vi "BELLA PW scan mode shot control shutter.vi"(8 "error in (no error)":errorcluster, 10 "PostScanRate":dbl=0.006 min=-9999999.0 max=9999999.0 format="%#_3f", 11 "ScanShotControl":bool) -> (0 "error out":errorcluster, 3 "delay D to set":dbl)   [LabVIEW 2020]
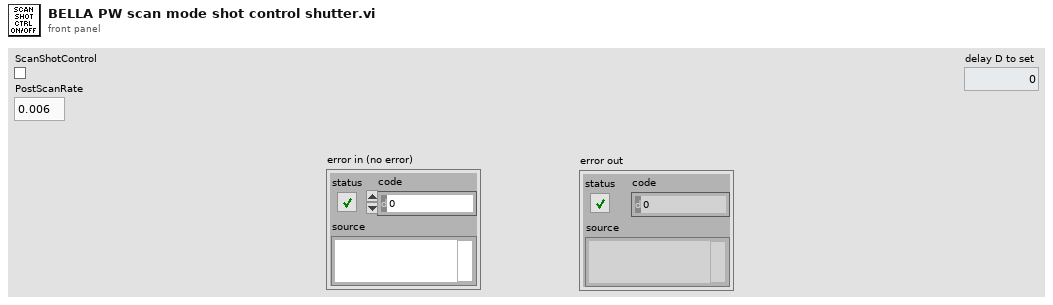
[diagram p1: front panel]
types:
  T1 = typedef "mysql_authentication.ctl" = cluster{"User":string, "Password":string, "Database":string}
  T2 = cluster{"Port":u16, "IP Address":string, "Authentication":T1}
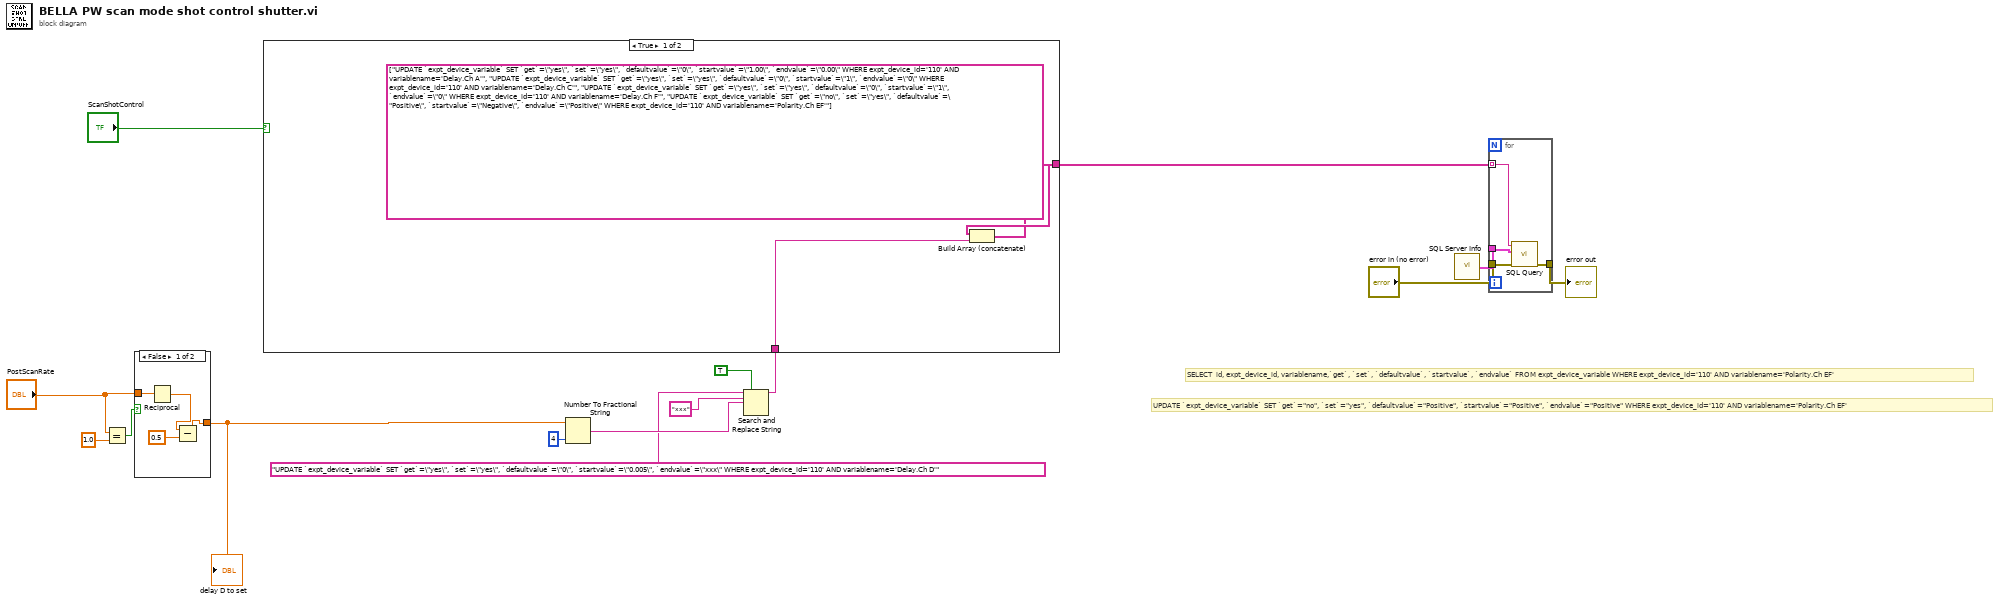
[diagram p0: block diagram]
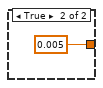
[diagram p2: hidden frame]
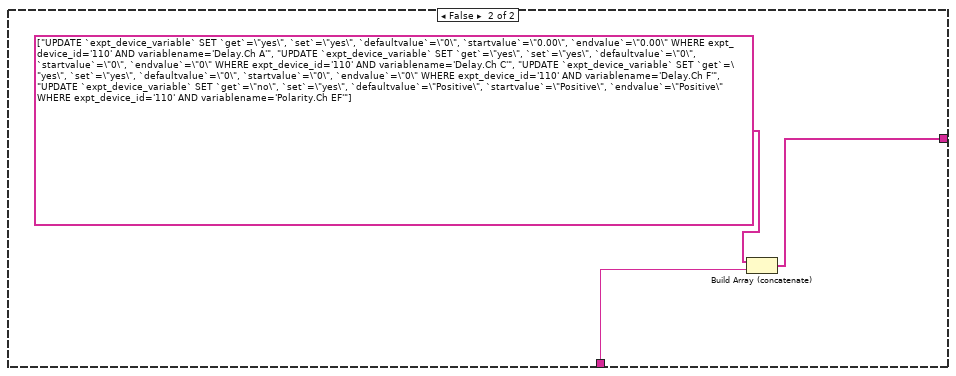
[diagram p3: hidden frame]
diagram:
  # "UPDATE `expt_device_variable` SET `get`=\"no\", `set`=\"yes\", `defaultvalue`=\"Positive\", `startvalue`=\"Positive\", `endvalue`=\"Positive\" WHERE expt_device_id='110' AND variablename='Polarity.Ch EF'"
  # "SELECT  id, expt_device_id, variablename,`get`, `set`, `defaultvalue`, `startvalue`, `endvalue` FROM expt_device_variable WHERE expt_device_id='110' AND variablename='Polarity.Ch EF'"
  n1 = Equal?(x="PostScanRate", y=1.0) -> (x = y?=w8:bool)
  n2 = case shown="False" w8 {
    tunnel: "PostScanRate" -> [w19 _]
    tunnel: [w16 0.005 ("y")] -> w5
    frame False {
      n3 = Reciprocal(x=w19) -> (1/x=w18:dbl)
      n4 = Subtract(x=w18, y=0.5) -> (x-y=w16:dbl)
    }
    frame True {
    }
  }
  "delay D to set" <- w5
  n5 = Number To Fractional String(number=w5, precision (6)=i16 4) -> (F-format string=w7:string)  [unwired: 2 in]
  n6 = Search and Replace String(replace all?=TRUE ("replace all? (F)"), input string="UPDATE `expt_device_variable` SET `get`=\"yes\", `set`=\"yes\", `defaultvalue`=\"0\", `startvalue`=\"0.005\", `endvalue`=\"xxx\" WHERE expt_device_id='110' AND variablename='Delay.Ch D'" ("Query"), search string="xxx", replace string=w7) -> (result string=w1:string)  [unwired: 4 in, 3 out]
  n7 = case shown="True" "ScanShotControl" {
    tunnel: [w22 w25] -> w14
    tunnel: w1 -> [w21 w24]
    frame True {
      n8 = Build Array (concatenate)(string[] ["UPDATE `expt_device_variable` SET `get`=\"yes\", `set`=\"yes\", `defaultvalue`=\"0\", `startvalue`=\"1.00\", `endvalue`=\"0.00\" WHERE expt_device_id='110' AND variablename='Delay.Ch A'", "UPDATE `expt_device_variable` SET `get`=\"yes\", `set`=\"yes\", `defaultvalue`=\"0\", `startvalue`=\"1\", `endvalue`=\"0\" WHERE expt_device_id='110' AND variablename='Delay.Ch C'", "UPDATE `expt_device_variable` SET `get`=\"yes\", `set`=\"yes\", `defaultvalue`=\"0\", `startvalue`=\"1\", `endvalue`=\"0\" WHERE expt_device_id='110' AND variablename='Delay.Ch F'", "UPDATE `expt_device_variable` SET `get`=\"no\", `set`=\"yes\", `defaultvalue`=\"Positive\", `startvalue`=\"Negative\", `endvalue`=\"Positive\" WHERE expt_device_id='110' AND variablename='Polarity.Ch EF'"], w21) -> (w22:string[])
    }
    frame False {
      n9 = Build Array (concatenate)(string[] ["UPDATE `expt_device_variable` SET `get`=\"yes\", `set`=\"yes\", `defaultvalue`=\"0\", `startvalue`=\"0.00\", `endvalue`=\"0.00\" WHERE expt_device_id='110' AND variablename='Delay.Ch A'", "UPDATE `expt_device_variable` SET `get`=\"yes\", `set`=\"yes\", `defaultvalue`=\"0\", `startvalue`=\"0\", `endvalue`=\"0\" WHERE expt_device_id='110' AND variablename='Delay.Ch C'", "UPDATE `expt_device_variable` SET `get`=\"yes\", `set`=\"yes\", `defaultvalue`=\"0\", `startvalue`=\"0\", `endvalue`=\"0\" WHERE expt_device_id='110' AND variablename='Delay.Ch F'", "UPDATE `expt_device_variable` SET `get`=\"no\", `set`=\"yes\", `defaultvalue`=\"Positive\", `startvalue`=\"Positive\", `endvalue`=\"Positive\" WHERE expt_device_id='110' AND variablename='Polarity.Ch EF'"], w24) -> (w25:string[])
    }
  }
  n10 = call "SQL Server Info.vi"() -> ("SQL Server Info"=w15:T2)
  n11 = for {
    tunnel: w14 -> [w30] mode=indexing
    tunnel: w15 -> [w29]
    tunnel: "error in (no error)" -> [w28]
    tunnel: [w27] -> w11
    n12 = call "SQL Query.vi"("error in (no error)"=w28, "SQL Server Info"=w29, "Query"=w30) -> ("error out"=w27:errorcluster)  [unwired: 7 in, 1 out]
  }
  "error out" <- w11
